vi "PostErrorToManager.vi"(8 "error in (no error)":errorcluster, 11 "CDependencyInspection in":refnum<class "CDependencyInspection.lvclass">) -> (0 "error out":errorcluster, 3 "CDependencyInspection out":refnum<class "CDependencyInspection.lvclass">)   [LabVIEW 2020, in "DependencyInspection.lvlib" / "CDependencyInspection.lvclass"]
uses:
  CDependencyInspection.lvclass
  ErrorManager/ErrorManager/ErrorType.ctl
  LabVIEWObjectInterfaces/IErrorManager/IErrorManager.lvclass
  ErrorManager/ErrorManager/ErrorManager.lvclass
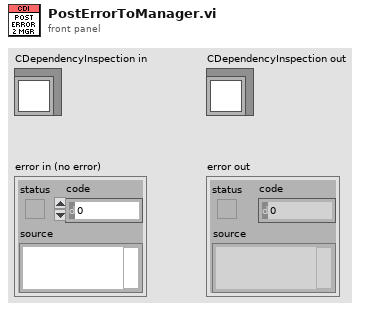
[diagram p1: front panel]
types:
  T1 = typedef "LabVIEWObjectInterfaces.lvlib/IErrorManager.lvclass/ErrorType.ctl" = enum16{"Info", "Warning", "Error"}
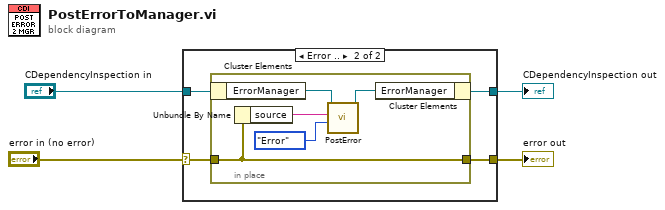
[diagram p0: block diagram]
diagram:
  n1 = case shown="Error .." "error in (no error)" {
    selector: "error in (no error)" -> [w5 w9]
    tunnel: "CDependencyInspection in" -> [w6 w10]
    tunnel: [w6 w8] -> w2
    tunnel: [w5 w7] -> w1
    frame No Error {
    }
    frame Error {
      n2 = in-place {
        in-place-border: w9 -> [w11]
        in-place-border: [w11] -> w7
        n3 = in-place-cluster #1(w10) -> ("ErrorManager"=w15:refnum<class "ErrorManager.lvclass">)
        n4 = Unbundle By Name(w11) -> ("source"=w13:string)
        n5 = call-dynamic "PostError.vi"("Type"=ErrorType."Error", "Message"=w13, "ErrorManager in"=w15) -> ("ErrorManager out"=w14:refnum<class "ErrorManager.lvclass">)  [unwired: 7 in, 1 out]
        n6 = in-place-cluster #1("ErrorManager"=w14) -> (w8:refnum<class "CDependencyInspection.lvclass">)
      }
    }
  }
  "error out" <- w1
  "CDependencyInspection out" <- w2
